vi "Main.vi"() -> ()   [LabVIEW 2013]
uses:
  <vilib>/Platform/storage/lvStorage.llb/_openFunction.ctl
  <vilib>/Platform/storage/lvStorage.llb/_openStorageWithRootAutoDetect.vi
  <vilib>/Platform/storage/lvStorage.llb/xStorage/xStorageSupp/ErrorOut.vi
  <vilib>/Platform/storage/lvStorage.llb/_queryPropPoly.vi
  <vilib>/Platform/storage/lvStorage.llb/_queryPropString.vi
  <vilib>/Platform/storage/lvStorage.llb/_queryGenericObjects.vi
  <vilib>/Platform/storage/lvStorage.llb/_loadAllWaveform.vi
  <vilib>/Platform/storage/Storage.llb/Get Object Info.vi
  <vilib>/Platform/storage/Storage.llb/__closeStorageFromObject.vi
  <vilib>/Platform/storage/lvStorage.llb/xStorage/Open Data Storage/Open Data Storage.xnode
  <vilib>/Platform/storage/lvStorage.llb/xStorage/Read Data/Read Data.xnode
  <vilib>/Platform/storage/lvStorage.llb/xStorage/Close Data Storage/Close Data Storage.xnode
panel:
  in  "Channel":enum16{"Right", "Left"}(ring)
  in  "Input File":path
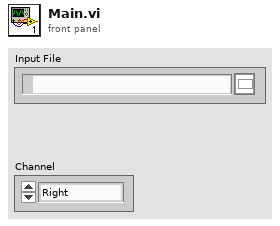
[diagram p1: front panel]
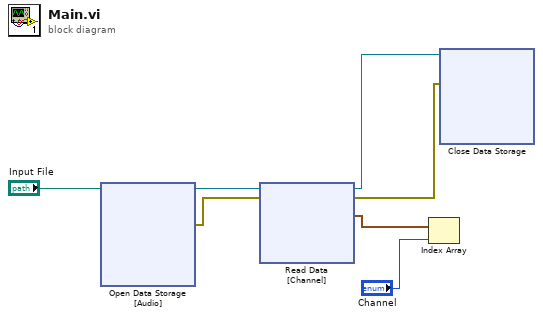
[diagram p0: block diagram]
diagram:
  n1 = xnode "Open Data Storage\n[Audio]"("file path"="Input File") -> ("storage refnum (file)"=w6:refnum<k20>, "error out"=w4:errorcluster)  [unwired: 4 in, 1 out]
  n2 = xnode "Read Data\n[Channel]"("storage refnum (file)"=w6, "error in"=w4) -> ("storage refnum (file) out"=w5:refnum<k20>, "error out"=w3:errorcluster, "Signal"=w2:waveform(dbl)[])  [unwired: 2 in, 1 out]
  n3 = Index Array(array=w2, index="Channel") -> ()  [unwired: 1 out]
  n4 = xnode "Close Data Storage\n"("storage refnum (file)"=w5, "error in (no error)"=w3) -> ()  [unwired: 2 out]
